vi "Convert RAWDATA.vi"(0 "UV-VIS in":refnum<class "UV-VIS.lvclass">, 1 "# of scan":i32, 2 "WCM_limits":T1, 3 "I channel seq IN":cluster{"BG":i32[], "Ie":i32[], "I0":i32[]}[](array[cluster]), 5 "I channel":i32[][](array[numeric]), 7 "WCM_values IN":sgl[](array[numeric]), 9 "II channel":i32[][](array[numeric]), 11 "error in (no error)":errorcluster, 12 "All?":bool=TRUE, 13 "WCM_correction":bool, 14 "II channel seq IN":cluster{"BG":i32[], "Ie":i32[], "I0":i32[]}[](array[cluster])) -> (4 "UV-VIS out":refnum<class "UV-VIS.lvclass">, 6 "I channel seq":cluster{"BG":i32[], "Ie":i32[], "I0":i32[]}[](array[cluster]), 8 "WCM_correction_coff":sgl[](array[numeric]), 10 "II channel seq":cluster{"BG":i32[], "Ie":i32[], "I0":i32[]}[](array[cluster]), 15 "error out":errorcluster)   [LabVIEW 2015]
uses:
  Detector.lvclass
  UV-VIS.lvclass
  dependecies/ControlsVIs/Clusters-def/Def_WCM_limits.ctl
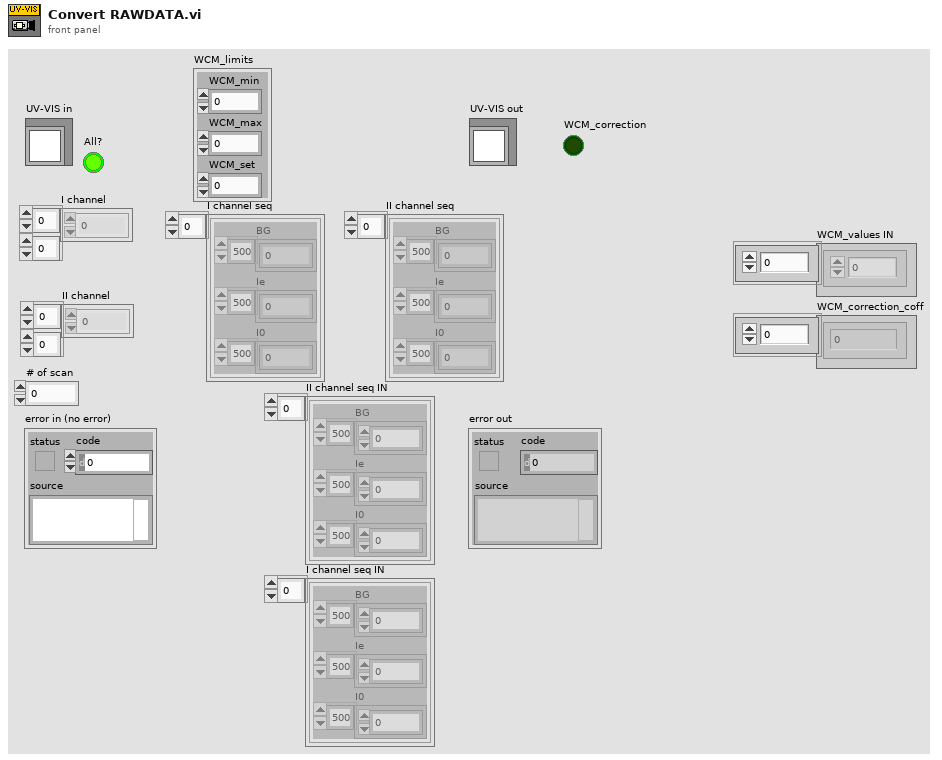
[diagram p1: front panel]
types:
  T1 = typedef "Def_WCM_limits.ctl" = cluster{"WCM_min":dbl, "WCM_max":dbl, "WCM_set":dbl}
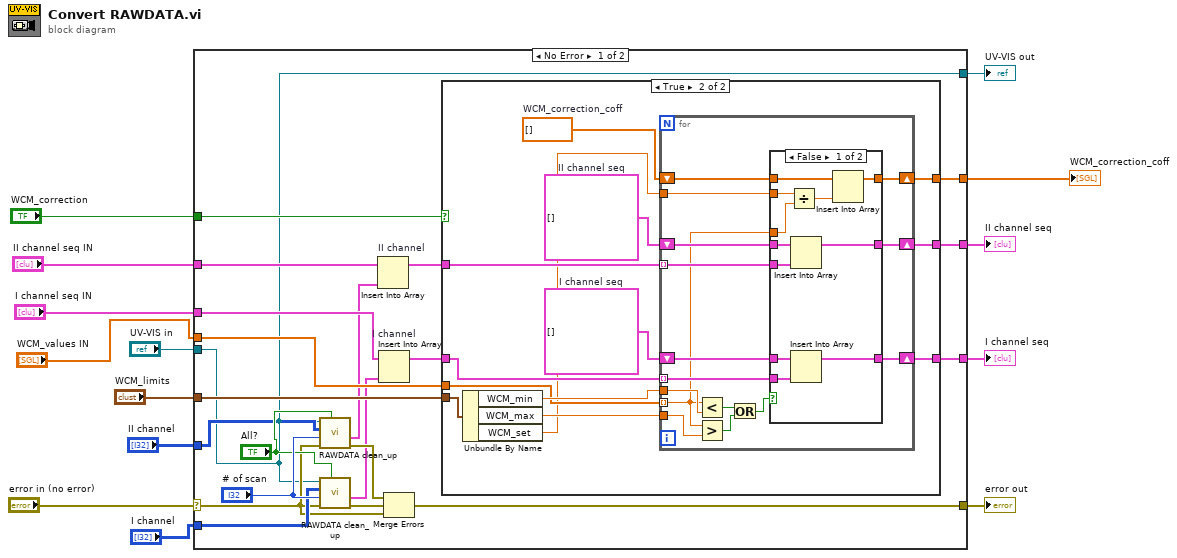
[diagram p0: block diagram]
diagram:
  n1 = case shown="No Error" "error in (no error)" {
    selector: "error in (no error)" -> [w18 w84]
    tunnel: [w15 w85] -> w13
    tunnel: "UV-VIS in" -> [w15 w85]
    tunnel: [w35 w84] -> w11
    tunnel: [w34 w83] -> w10
    tunnel: [w32 w82] -> w9
    tunnel: "II channel seq IN" -> [w30 w83]
    tunnel: "I channel seq IN" -> [w29 w82]
    tunnel: [w28 w81] -> w6
    tunnel: "WCM_values IN" -> [w27 w81]
    tunnel: "I channel" -> [w19 _]
    tunnel: "II channel" -> [w17 _]
    tunnel: "WCM_correction" -> [w26 _]
    tunnel: "WCM_limits" -> [w25 _]
    frame No Error {
      n2 = call "RAWDATA clean_up.vi"("All?"="All?", "error in (no error)"=w18, "# of scan"="# of scan", "channel"=w17, "Detector in"=w15) -> ("error out"=w21:errorcluster, "channel seq"=w16:cluster{"BG":i32[], "Ie":i32[], "I0":i32[]}[])  [unwired: 4 in, 1 out]
      n3 = call "RAWDATA clean_up.vi"("All?"="All?", "error in (no error)"=w18, "# of scan"="# of scan", "channel"=w19, "Detector in"=w15) -> ("error out"=w22:errorcluster, "channel seq"=w20:cluster{"BG":i32[], "Ie":i32[], "I0":i32[]}[])  [unwired: 4 in, 1 out]
      n4 = Insert Into Array "II channel"(array=w30, new element=w16) -> (w33:cluster{"BG":i32[], "Ie":i32[], "I0":i32[]}[])  [unwired: 1 in]
      n5 = Insert Into Array "I channel"(array=w29, new element=w20) -> (w31:cluster{"BG":i32[], "Ie":i32[], "I0":i32[]}[])  [unwired: 1 in]
      n6 = Merge Errors(w21, w22, w18) -> (w35:errorcluster)
      n7 = case shown="True" w26 {
        tunnel: [w38 w43] -> w34
        tunnel: w33 -> [w38 w45]
        tunnel: [w37 w44] -> w32
        tunnel: w31 -> [w37 w46]
        tunnel: [w36 w42] -> w28
        tunnel: w27 -> [w36 w41]
        tunnel: w25 -> [_ w40]
        frame False {
        }
        frame True {
          w50 = cluster{"BG":i32[], "Ie":i32[], "I0":i32[]}[] []  # II channel seq
          w51 = cluster{"BG":i32[], "Ie":i32[], "I0":i32[]}[] []  # I channel seq
          w47 = sgl[] []  # WCM_correction_coff
          n8 = Unbundle By Name(w40) -> ("WCM_min"=w49:dbl, "WCM_max"=w48:dbl, "WCM_set"=w39:dbl)
          n9 = for {
            tunnel: w48 -> [w65]
            tunnel: w49 -> [w66]
            shift-right: [w63] -> w42
            shift-left: w47 -> [w64]
            shift-right: [w57] -> w43
            shift-left: w50 -> [w56]
            shift-right: [w58] -> w44
            shift-left: w51 -> [w59]
            tunnel: w46 -> [w55] mode=indexing
            tunnel: w45 -> [w54] mode=indexing
            tunnel: w41 -> [w52] mode=indexing
            tunnel: w39 -> [w53]
            n10 = Less?(x=w52, y=w66) -> (x < y?=w62:bool)
            n11 = Greater?(x=w52, y=w65) -> (0:w61:bool)
            n12 = Or(x=w62, y=w61) -> (x .or. y?=w60:bool)
            n13 = case shown="False" w60 {
              tunnel: [w76 w80] -> w63
              tunnel: w64 -> [w77 w80]
              tunnel: w59 -> [w75 w79]
              tunnel: [w74 w79] -> w58
              tunnel: [w72 w78] -> w57
              tunnel: w56 -> [w73 w78]
              tunnel: w55 -> [w71 _]
              tunnel: w54 -> [w70 _]
              tunnel: w53 -> [w69 _]
              tunnel: w52 -> [w68 _]
              frame False {
                n14 = Divide(x=w69, y=w68) -> (x/y=w67:dbl)
                n15 = Insert Into Array(array=w73, new element=w70) -> (w72:cluster{"BG":i32[], "Ie":i32[], "I0":i32[]}[])  [unwired: 1 in]
                n16 = Insert Into Array(array=w75, new element=w71) -> (w74:cluster{"BG":i32[], "Ie":i32[], "I0":i32[]}[])  [unwired: 1 in]
                n17 = Insert Into Array(array=w77, new element=w67) -> (w76:sgl[])  [unwired: 1 in]
              }
              frame True {
              }
            }
          }
        }
      }
    }
    frame Error {
    }
  }
  "error out" <- w11
  "UV-VIS out" <- w13
  "II channel seq" <- w10
  "I channel seq" <- w9
  "WCM_correction_coff" <- w6
